vi "ex6-3.vi"   [LabVIEW 2013]
uses:
  <vilib>/NXT/Dual Mode Library/Sensors/EV3_Color_Color.vi
  <vilib>/NXT/Dual Mode Library/Display/drawNumber.vi
  <vilib>/NXT/NXTIO Xnodes/NXTIONodeSubVIs/LEGOMoveAllMotors.vi
  <vilib>/NXT/NXTIO Xnodes/NXTIONodeSubVIs/LEGOStopAllMotors.vi
  <vilib>/NXT/Subs/LVHSConnector.ctl
  <vilib>/NXT/NXTIO Xnodes/NXTIOXNode/NXTIO.xnode
  <vilib>/NXT/LegoClasses/BrickReference/BrickReference.lvclass
types:
  T1 = typedef "ColorSensorColors.ctl" = enum16{"No Color", "Black", "Blue", "Green", "Yellow", "Red", "White", "Brown"}
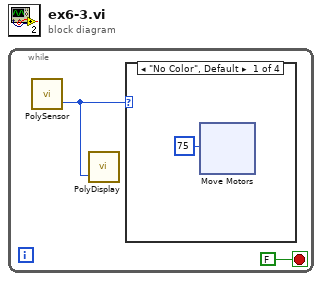
[diagram p0: block diagram]
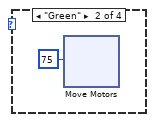
[diagram p2: hidden frame]
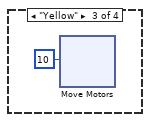
[diagram p3: hidden frame]
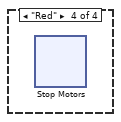
[diagram p4: hidden frame]
diagram:
  n1 = while {
    stop <- FALSE stop-if-true
    n2 = call-poly <vilib>:"PolySensor.vi"() -> ("Detected Color"=w1:T1)  [unwired: 3 in, 1 out]
    n3 = call-poly <vilib>:"PolyDisplay.vi"("number"=w1) -> ()  [unwired: 3 in, 1 out]
    n4 = case shown="\"No Color\", Default" w1 {
      frame "No Color", Default {
        n5 = xnode "Move Motors"("Power/Speed 1"=i8 75) -> ()  [unwired: 2 in, 1 out]
      }
      frame "Green" {
        n6 = xnode "Move Motors"("Power/Speed 1"=i8 75) -> ()  [unwired: 2 in, 1 out]
      }
      frame "Yellow" {
        n7 = xnode "Move Motors"("Power/Speed 1"=i8 10) -> ()  [unwired: 2 in, 1 out]
      }
      frame "Red" {
        n8 = xnode "Stop Motors"() -> ()  [unwired: 2 in, 1 out]
      }
    }
  }
